vi "HNE Page Manager (Init).vi"(3 "error in (no error)":errorcluster, 4 "Max page history length":i32, 5 "Initial Page":string) -> (0 "error out":errorcluster)   [LabVIEW 2013]
doc: "This VI initializes the HMI Naviagtion Engine (HNE) by specifying the length for the pages history and writing to the Page Manager the name of the first page that will be displayed."
uses:
  _SubVIs/TypeDefs/Page Operation.ctl
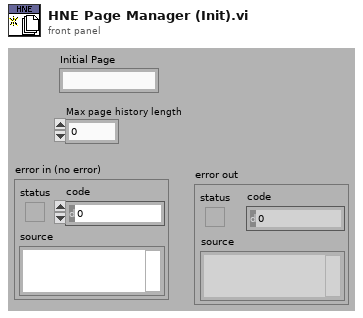
[diagram p1: front panel]
types:
  T1 = typedef "Page Operation.ctl" = enum16{"Init", "Set Next", "Get Next", "Back"}
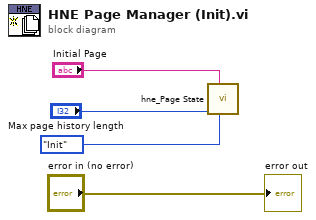
[diagram p0: block diagram]
diagram:
  n1 = call "hne_Page State.vi"("Page Operation"=Page_Operation."Init", "Initial Page"="Initial Page", "Max page history length"="Max page history length") -> ()  [unwired: 1 in, 8 out]
  "error out" <- "error in (no error)"
